vi "Voice Report.vi"(5 "Report Enable":T1, 7 "Reporting Interval (s)":dbl=10.0, 8 "Data":dbl, 10 "Description":string="Speed") -> ()   [LabVIEW 2014]
uses:
  Controls/Enable Voice Reporting.ctl
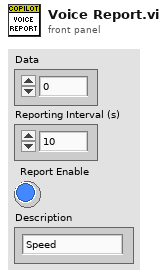
[diagram p1: front panel]
types:
  T1 = typedef "Enable Voice Reporting.ctl" = bool
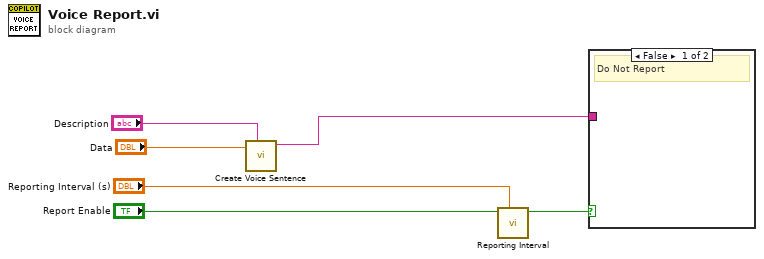
[diagram p0: block diagram]
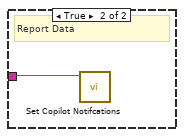
[diagram p2: hidden frame]
diagram:
  n1 = call "Create Voice Sentence.vi"("Description"="Description", "Number"="Data") -> ("Voice Reporting Sentence"=w3:string)  [unwired: 9 in]
  n2 = call "Reporting Interval.vi"("Reporting Interval (s)"="Reporting Interval (s)", "Report Enable"="Report Enable") -> ("Report Data"=w6:T1)  [unwired: 9 in]
  n3 = case shown="False" w6 {
    tunnel: w3 -> [_ w7]
    frame False {
      # "Do Not Report"
    }
    frame True {
      # "Report Data"
      n4 = call "Set Copilot Notifcations.vi"("Notification"=w7) -> ()  [unwired: 10 in, 1 out]
    }
  }
